vi "Keithley24XX_Ramp_Prog.vi"() -> ()   [LabVIEW 2019]
uses:
  <instrlib>/Keithley 24XX/Public/Data/Read (Single Point).vi
  <instrlib>/Keithley 24XX/Keithley 24XX.lvlib
panel:
  in  "Stop Program":bool
  in  "Delay Time (s)":dbl=0.5 format="%#_13g"
  in  "Compliance  Level (0.1)":dbl=1e-07
  in  "Gate Voltage Setpoint":dbl
  in  "Step Size (V)":dbl=0.1
  in  "Run":bool
  out "Internal Measurement Time":u32
  out "Voltage vs N : XYGraph 3":cluster{"X":dbl[], "Y":dbl[]}[](graph)
  out "Gate\nVoltage":sgl
  out "Status":sgl
  out "Leakage \nCurrent":sgl
  out "I_leak vs N : XYGraph 2":cluster{"X":dbl[], "Y":dbl[]}[](graph)
  in  "Reset (Note, you  may need to set TRUE to get readout working! \nDon't use TRUE when measuring a device!). This program should loop\nthe voltage from the sourcemeter from 0V to 0.5V then jump to 0V and repeat.":bool
  in  "Serial Configuration":T1={"Baud Rate"=9600, "Parity"=0, "Data Bits"=8, "Stop Bits"=10, "Flow Control"=0} {"Flow Control" items=["None", "XON/XOFF", "RTS/CTS", "XON/XOFF & RTS/CTS", "DTR/DSR", "XON/XOFF & DTR/DSR"]; "Stop Bits" items=["1.0"=10, "1.5"=15, "2.0"=20]; "Data Bits" items=["7"=7, "8"=8]; "Parity" items=["None", "Odd", "Even", "Mark", "Space"]; "Baud Rate" items=["300"=300, "600"=600, "1200"=1200, "2400"=2400, "4800"=4800, "9600"=9600, "19200"=19200]}
  in  "Keithley24XX VISA resource name":refnum<visa-resource-name>="GPIB0::21::INSTR" caption="Keithley 24XX VISA resource name"
  # "Sub-program to change\ngate voltage setpoint.\nClick run to increment \nto setpoint."
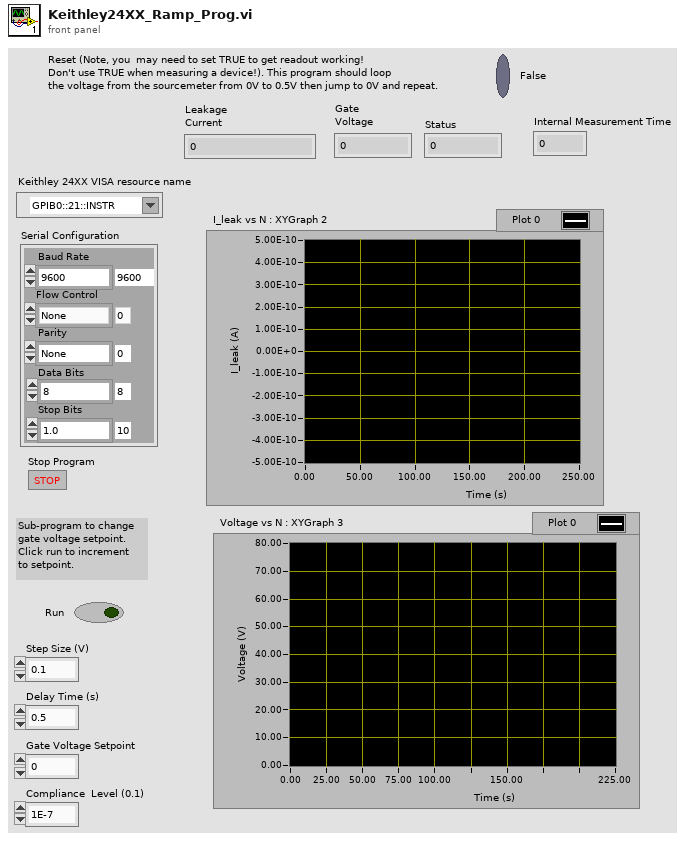
[diagram p1: front panel]
types:
  T1 = cluster{"Baud Rate":u32, "Parity":u16, "Data Bits":u16, "Stop Bits":u16, "Flow Control":u16}
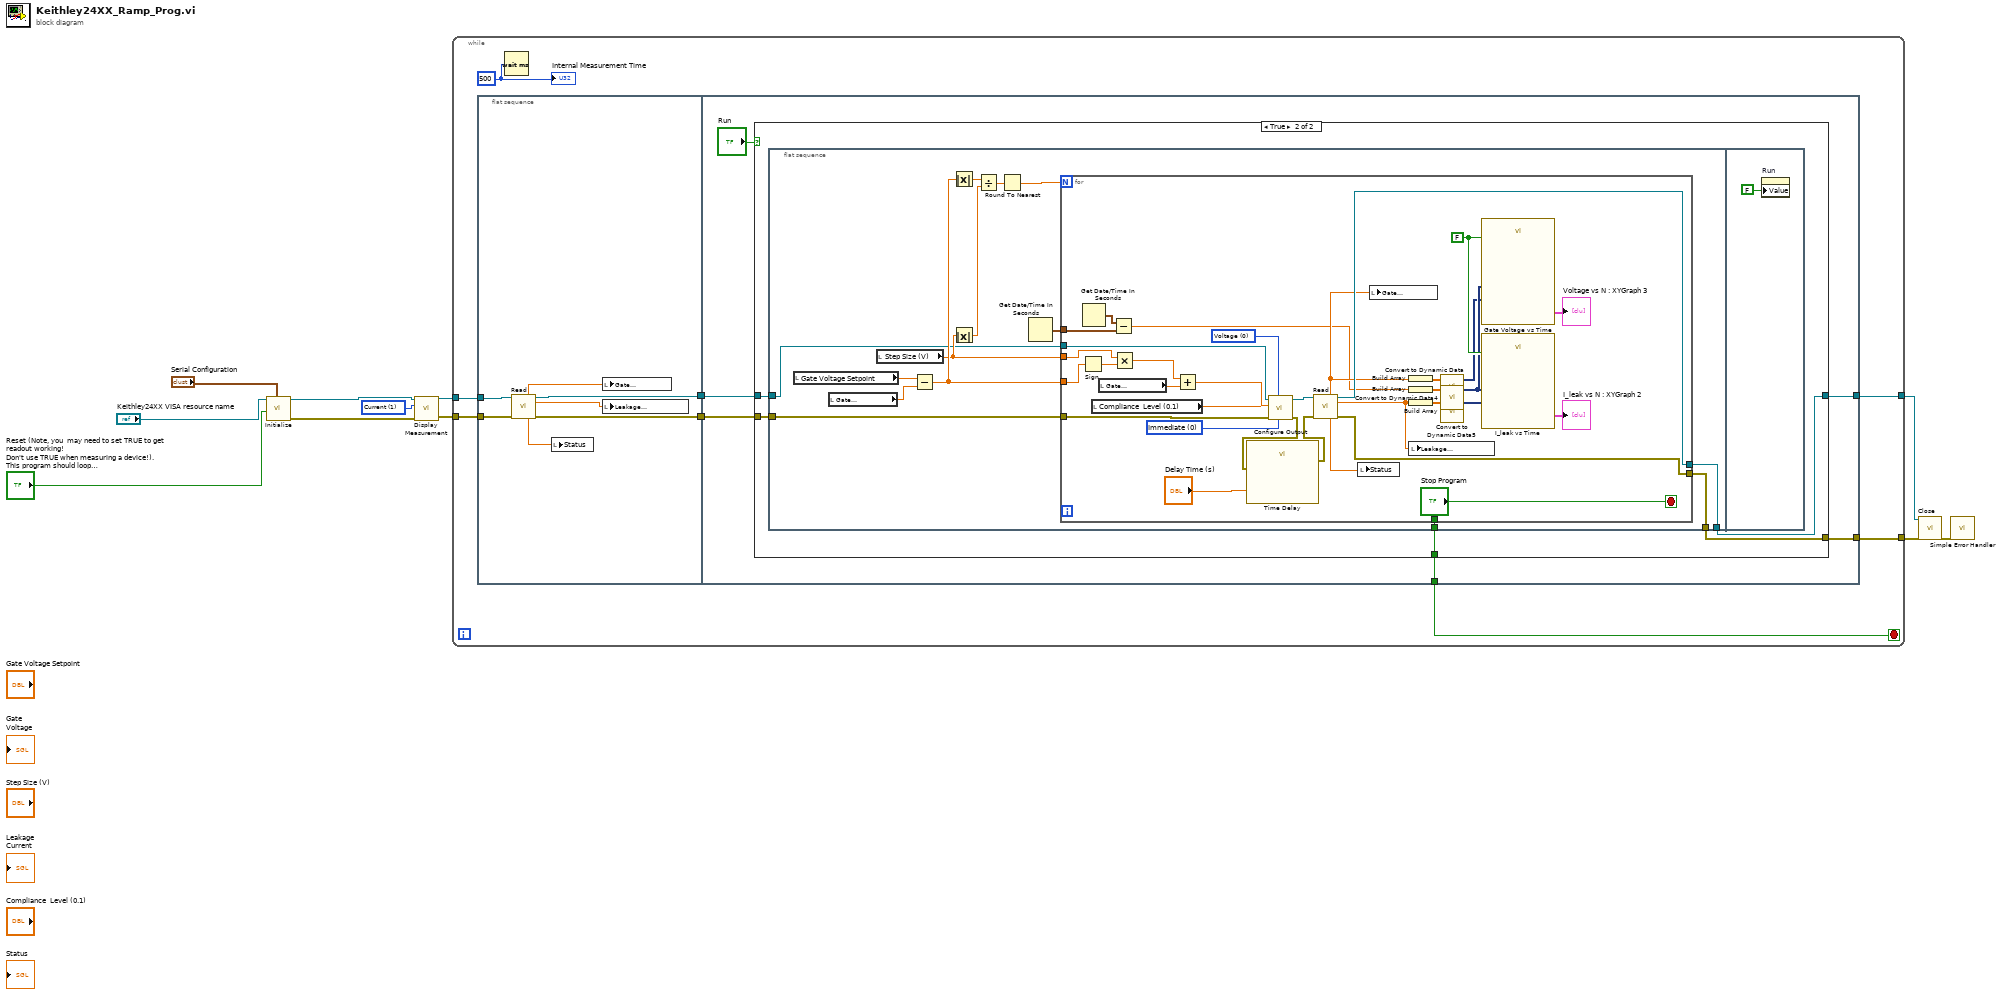
[diagram p0: block diagram]
diagram:
  w8 = u16 1 items=["Voltage", "Current", "Resistance"] ("Displayed Measurement (0: Voltage)")
  n1 = call <instrlib>:"Initialize.vi"("Serial Configuration"="Serial Configuration", "Reset (True)"="Reset (Note, you  may need to set TRUE to get readout working! \nDon't use TRUE when measuring a device!). This program should loop\nthe voltage from the sourcemeter from 0V to 0.5V then jump to 0V and repeat.", "VISA resource name"="Keithley24XX VISA resource name") -> ("error out"=w6:errorcluster, "VISA resource name out"=w7:refnum<visa-resource-name>)  [unwired: 7 in]
  n2 = call <instrlib>:"Display Measurement.vi"("error in (no error)"=w6, "Displayed Measurement (0: Voltage)"=w8, "VISA resource name"=w7) -> ("error out"=w4:errorcluster, "VISA resource name out"=w5:refnum<visa-resource-name>)  [unwired: 7 in]
  n3 = while {
    tunnel: w5 -> [w18]
    tunnel: w4 -> [w17]
    tunnel: [w14] -> w3
    tunnel: [w13] -> w2
    stop <- w12 stop-if-true
    w19 = u32 500 ("milliseconds to wait")
    n4 = flat-sequence {
      tunnel: w18 -> [w26]
      tunnel: w17 -> [w25]
      tunnel: [w21] -> w16
      tunnel: [w20] -> w15
      tunnel: w16 -> [w31]
      tunnel: w15 -> [w30]
      tunnel: [w29] -> w14
      tunnel: [w28] -> w13
      tunnel: [w27] -> w12
      frame #0 {
        n5 = call-poly <instrlib>:"Read.vi"("VISA resource name"=w26, "error in (no error)"=w25) -> ("Voltage"=w22:sgl, "VISA resource name out"=w21:refnum<visa-resource-name>, "Current"=w23:sgl, "Status"=w24:sgl, "error out"=w20:errorcluster)  [unwired: 7 in, 2 out]
        n6 = local write "Status"(w24) -> ()
        n7 = local write "Gate\nVoltage"(w22) -> ()
        n8 = local write "Leakage \nCurrent"(w23) -> ()
      }
      frame #1 {
        n9 = case shown="True" "Run" {
          tunnel: w31 -> [w34 w39]
          tunnel: w30 -> [w33 w38]
          tunnel: [w34 w37] -> w29
          tunnel: [w33 w36] -> w28
          tunnel: [_ w35] -> w27
          frame False {
          }
          frame True {
            n10 = flat-sequence {
              tunnel: w39 -> [w45]
              tunnel: w38 -> [w44]
              tunnel: [w43] -> w37
              tunnel: [w42] -> w36
              tunnel: [w40] -> w35
              frame #0 {
                n11 = local read "Gate Voltage Setpoint"() -> (w49:dbl)
                n12 = local read "Gate\nVoltage"() -> (w50:sgl)
                n13 = local read "Step Size (V)"() -> (w46:dbl)
                n14 = Subtract(x=w49, y=w50) -> (x-y=w51:dbl)
                n15 = Absolute Value(x=w51) -> (abs(x)=w48:dbl)
                n16 = Absolute Value(x=w46) -> (abs(x)=w47:dbl)
                n17 = Divide(x=w48, y=w47) -> (x/y=w53:dbl)
                n18 = Round To Nearest(number=w53) -> (nearest integer value=w52:dbl)
                n19 = Get Date/Time In Seconds() -> (seconds since 1Jan1904=w41:timestamp)
                n20 = for {
                  N: w52 -> [_]
                  tunnel: w51 -> [w86]
                  tunnel: w46 -> [w85]
                  tunnel: w45 -> [w78]
                  tunnel: w44 -> [w77]
                  tunnel: [w73] -> w43
                  tunnel: [w72] -> w42
                  tunnel: w41 -> [w68]
                  tunnel: ["Stop Program"] -> w40
                  stop <- "Stop Program" stop-if-true
                  w64 = FALSE ("Reset")
                  w80 = u16 0 items=["Immediate", "Triggered"] ("Output Type  (0: Immediate)")
                  w81 = u16 0 items=["Voltage", "Current"] ("Source Mode  (0: Voltage)")
                  n21 = Sign(1:w86) -> (0:w84:dbl)
                  n22 = Get Date/Time In Seconds() -> (seconds since 1Jan1904=w69:timestamp)
                  n23 = local read "Compliance  Level (0.1)"() -> (w79:dbl)
                  n24 = local read "Gate\nVoltage"() -> (w58:sgl)
                  n25 = Subtract(x=w69, y=w68) -> (x-y=w67:dbl)
                  n26 = Multiply(x=w85, y=w84) -> (x*y=w83:dbl)
                  n27 = Add(x=w83, y=w58) -> (x+y=w82:dbl)
                  n28 = call <instrlib>:"Configure Output.vi"("Output Type  (0: Immediate)"=w80, "Source Mode  (0: Voltage)"=w81, "error in (no error)"=w77, "Compliance  Level (0.1)"=w79, "Output Level (0)"=w82, "VISA resource name"=w78) -> ("error out"=w57:errorcluster, "VISA resource name out"=w74:refnum<visa-resource-name>)  [unwired: 4 in]
                  n29 = call "Time Delay"("error in (no error)"=w57, "Delay Time (s)"="Delay Time (s)") -> ("error out"=w56:errorcluster)  [unwired: 9 in]
                  n30 = call-poly <instrlib>:"Read.vi"("VISA resource name"=w74, "error in (no error)"=w56) -> ("Voltage"=w71:sgl, "VISA resource name out"=w73:refnum<visa-resource-name>, "Current"=w70:sgl, "Status"=w75:sgl, "error out"=w72:errorcluster)  [unwired: 7 in, 2 out]
                  n31 = local write "Status"(w75) -> ()
                  n32 = local write "Gate\nVoltage"(w71) -> ()
                  n33 = Build Array(w71) -> (w62:sgl[])
                  n34 = Build Array(w67) -> (w66:dbl[])
                  n35 = Build Array(w70) -> (w65:sgl[])
                  n36 = local write "Leakage \nCurrent"(w70) -> ()
                  n37 = call "Convert to Dynamic Data"("Array"=w62) -> ("Dynamic Data Type"=w61:dynamicdata)  [unwired: 3 in]
                  n38 = call "Convert to Dynamic Data4"("Array"=w66) -> ("Dynamic Data Type"=w63:dynamicdata)  [unwired: 3 in]
                  n39 = call "Convert to Dynamic Data5"("Array"=w65) -> ("Dynamic Data Type"=w76:dynamicdata)  [unwired: 3 in]
                  n40 = call "Gate Voltage vs Time"("Reset"=w64, "Y Input"=w61, "X Input"=w63) -> ("XY Graph"=→"Voltage vs N : XYGraph 3":cluster{"X":dbl[], "Y":dbl[]}[])  [unwired: 7 in, 1 out]
                  n41 = call "I_leak vs Time"("Reset"=w64, "Y Input"=w76, "X Input"=w63) -> ("XY Graph"=→"I_leak vs N : XYGraph 2":cluster{"X":dbl[], "Y":dbl[]}[])  [unwired: 7 in, 1 out]
                }
              }
              frame #1 {
                n42 = property on="Run" class="Bool (strict)"("Value"=FALSE ("Run")) -> ()  [unwired: 2 in, 2 out]
              }
            }
          }
        }
      }
    }
    n43 = Wait (ms)(milliseconds to wait=w19) -> ()  [unwired: 1 out]
    "Internal Measurement Time" <- w19
  }
  n44 = call <instrlib>:"Close.vi"("error in (no error)"=w2, "VISA resource name"=w3) -> ("error out"=w9:errorcluster)  [unwired: 9 in]
  n45 = call <vilib>:"Simple Error Handler.vi"("error in (no error)"=w9) -> ()  [unwired: 4 in, 5 out]
